vi "Do Attacked.vi"(7 "Team In":refnum<class "Team.lvclass">, 10 "Attackers":i32[](array[numeric]), 11 "Square":refnum<class "Square.lvclass">) -> (5 "Team out":refnum<class "Team.lvclass">)   [LabVIEW 2020, in "SquareBattle.lvlib" / "Square.lvclass"]
uses:
  Square.lvclass
  Square.lvclass/Square.ctl
  Team/Team.lvclass
  Team Stats.ctl
  SquareBattle.lvlib
  Attacked Info.ctl
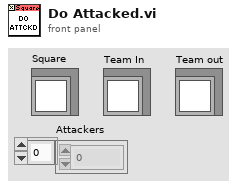
[diagram p1: front panel]
types:
  T1 = typedef "SquareBattle.lvlib/Attacked Info.ctl" = cluster{"Attackers":i32[]}
  T2 = typedef "SquareBattle.lvlib/Team Stats.ctl" = cluster{"Active":i32, "Generated":i32, "Kills":i32, "Eliminated":i32, "Collided":i32}
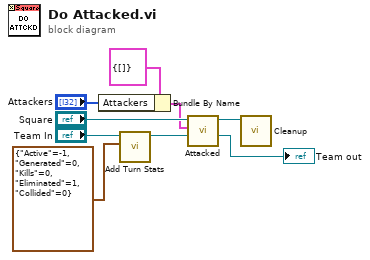
[diagram p0: block diagram]
diagram:
  n1 = Bundle By Name(cluster=T1 {"Attackers"=[]} ("Attacked Info"), "Attackers"="Attackers") -> (w1:T1)
  n2 = call "Add Turn Stats.vi"("Team Stats"=T2 {"Active"=-1, "Generated"=0, "Kills"=0, "Eliminated"=1, "Collided"=0}, "Team in"="Team In") -> ("Team out"=w6:refnum<class "Team.lvclass">)  [unwired: 9 in]
  n3 = call-dynamic "Attacked.vi"("Team In"=w6, "Attackers"=w1, "Square in"="Square") -> ("Team"=→"Team out":refnum<class "Team.lvclass">, "Square out"=w4:refnum<class "Square.lvclass">)  [unwired: 7 in]
  n4 = call-dynamic "Cleanup.vi"("Square"=w4) -> ()  [unwired: 11 in]
